vi "Convert RectifierListData to Arrays.vi"(0 "MulticolumnListbox in":refnum<vi>, 11 "error in (no error)":errorcluster) -> (2 "Fwd Tm":dbl[](array[numeric]), 3 "Rev Tm":dbl[](array[numeric]), 4 "Left Amps":dbl[](array[numeric]), 6 "Right Amps":dbl[](array[numeric]), 8 "Left AmpMins":dbl[](array[numeric]), 10 "Right Amp Min":dbl[](array[numeric]), 13 "Fwd Off Tm":dbl[](array[numeric]), 14 "Rev Off Tm":dbl[](array[numeric]), 15 "error out":errorcluster)   [LabVIEW 2019]
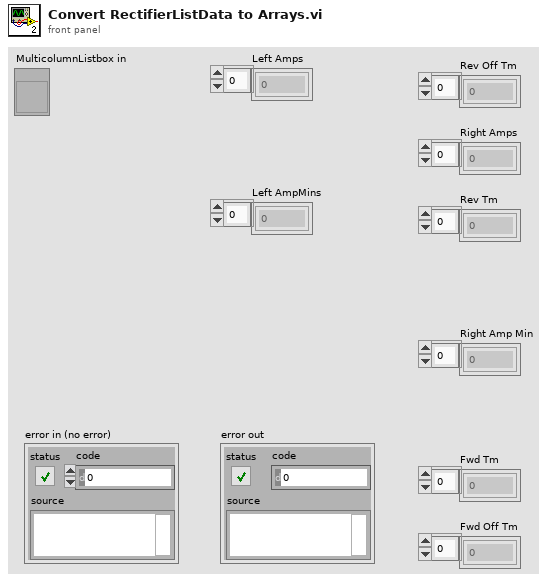
[diagram p1: front panel]
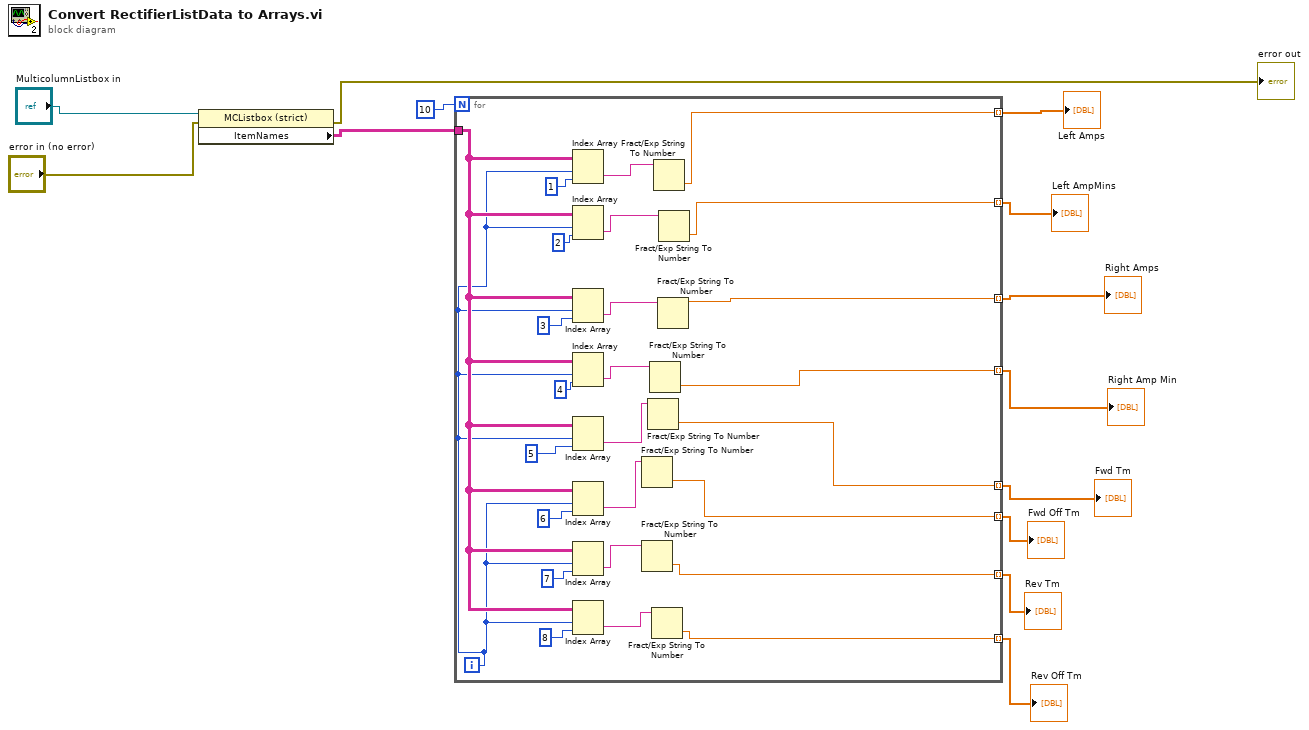
[diagram p0: block diagram]
diagram:
  n1 = property class="MCListbox (strict)"(reference="MulticolumnListbox in", error in="error in (no error)") -> (error out=→"error out":errorcluster, "ItemNames"=w12:string[][])  [unwired: 1 out]
  n2 = for {
    N: 10 -> [_]
    tunnel: w12 -> [w30]
    tunnel: [w18] -> w4 mode=indexing
    tunnel: [w15] -> w5 mode=indexing
    tunnel: [w17] -> w6 mode=indexing
    tunnel: [w14] -> w7 mode=indexing
    tunnel: [w22] -> w8 mode=indexing
    tunnel: [w21] -> w9 mode=indexing
    tunnel: [w20] -> w10 mode=indexing
    tunnel: [w19] -> w11 mode=indexing
    i -> [w16]
    n3 = Index Array(array=w30, index (row)=w16, index (col)=1 ("disabled index (col)")) -> (element=w38:string)
    n4 = Index Array(array=w30, index (row)=w16, index (col)=2 ("disabled index (col)")) -> (element=w29:string)
    n5 = Index Array(array=w30, index (row)=w16, index (col)=3 ("disabled index (col)")) -> (element=w28:string)
    n6 = Index Array(array=w30, index (row)=w16, index (col)=4 ("disabled index (col)")) -> (element=w27:string)
    n7 = Index Array(array=w30, index (row)=w16, index (col)=5 ("disabled index (col)")) -> (element=w26:string)
    n8 = Index Array(array=w30, index (row)=w16, index (col)=6 ("disabled index (col)")) -> (element=w25:string)
    n9 = Index Array(array=w30, index (row)=w16, index (col)=7 ("disabled index (col)")) -> (element=w24:string)
    n10 = Index Array(array=w30, index (row)=w16, index (col)=8 ("disabled index (col)")) -> (element=w23:string)
    n11 = Fract/Exp String To Number(string=w25) -> (number=w21:dbl)  [unwired: 3 in, 1 out]
    n12 = Fract/Exp String To Number(string=w24) -> (number=w20:dbl)  [unwired: 3 in, 1 out]
    n13 = Fract/Exp String To Number(string=w26) -> (number=w22:dbl)  [unwired: 3 in, 1 out]
    n14 = Fract/Exp String To Number(string=w27) -> (number=w14:dbl)  [unwired: 3 in, 1 out]
    n15 = Fract/Exp String To Number(string=w23) -> (number=w19:dbl)  [unwired: 3 in, 1 out]
    n16 = Fract/Exp String To Number(string=w38) -> (number=w18:dbl)  [unwired: 3 in, 1 out]
    n17 = Fract/Exp String To Number(string=w28) -> (number=w17:dbl)  [unwired: 3 in, 1 out]
    n18 = Fract/Exp String To Number(string=w29) -> (number=w15:dbl)  [unwired: 3 in, 1 out]
  }
  "Rev Off Tm" <- w11
  "Rev Tm" <- w10
  "Fwd Off Tm" <- w9
  "Fwd Tm" <- w8
  "Right Amp Min" <- w7
  "Right Amps" <- w6
  "Left AmpMins" <- w5
  "Left Amps" <- w4
